vi "Get Master From List.vi"(3 "error in":errorcluster, 4 "Del From List?":bool, 5 "Device List in":refnum<class "Device.lvclass">[](array[class])) -> (0 "error out":errorcluster, 1 "Master Device":refnum<class "Master Device.lvclass">, 2 "Device List out":refnum<class "Device.lvclass">[](array[class]))   [LabVIEW 2013]
uses:
  Device/Device.lvclass
  Master Device/Master Device.lvclass
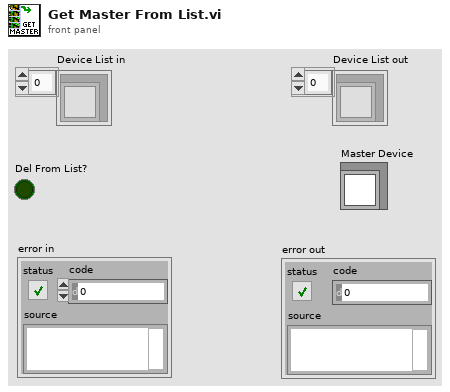
[diagram p1: front panel]
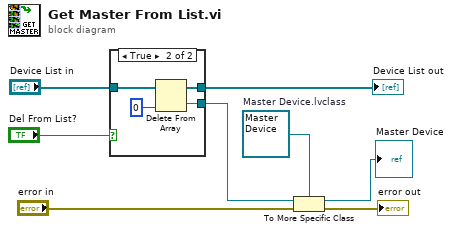
[diagram p0: block diagram]
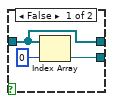
[diagram p2: hidden frame]
diagram:
  w7 = refnum<class "Master Device.lvclass"> refnum  # Master Device.lvclass
  n1 = case shown="True" "Del From List?" {
    tunnel: "Device List in" -> [w10 w15]
    tunnel: [w11 w13] -> w6
    tunnel: [w10 w14] -> w1
    frame False {
      n2 = Index Array(array=w10, index=0) -> (element=w11:refnum<class "Device.lvclass">)
    }
    frame True {
      n3 = Delete From Array(array=w15, index=0) -> (deleted portion=w13:refnum<class "Device.lvclass">, array with subset deleted=w14:refnum<class "Device.lvclass">[])  [unwired: 1 in]
    }
  }
  "Device List out" <- w1
  n4 = To More Specific Class(target class=w7, reference=w6, error in="error in") -> (specific class reference=→"Master Device":refnum<class "Master Device.lvclass">, error out=→"error out":errorcluster)
